vi "dirtyVision.vi"(11 "Plugin Info":T1) -> ()   [LabVIEW 2016]
uses:
  General/CorePluginInfo.ctl
panel:
  out "Frame Rate":dbl
  out "Image Out":T2(plugin-control)
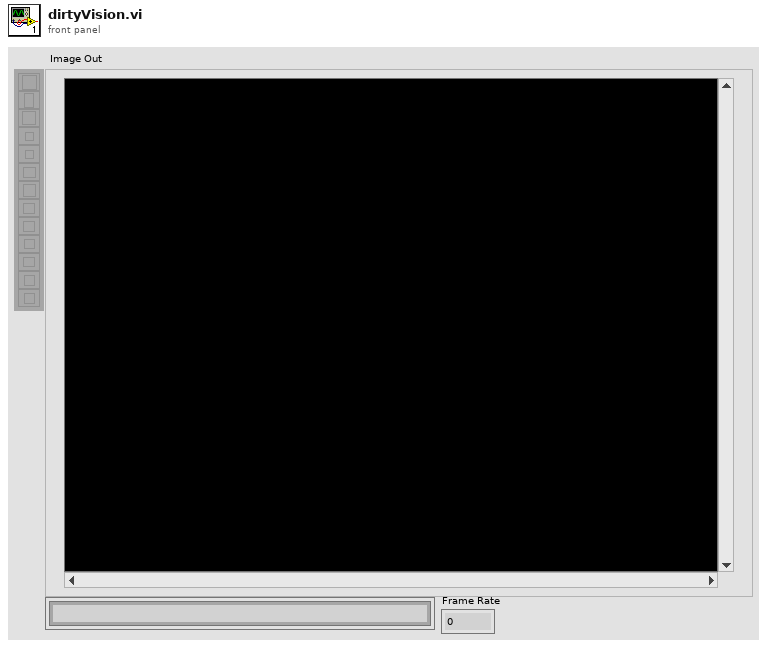
[diagram p1: front panel]
types:
  T1 = typedef "CorePluginInfo.ctl" = cluster{"Notifiers":cluster{"Robot IP Notifier":refnum<notifier>, "Window Mode Notifier":refnum<notifier>, "Stop Notifier":refnum<notifier>}}
  T2 = typedef "IMAQ Image.ctl" = refnum<image>
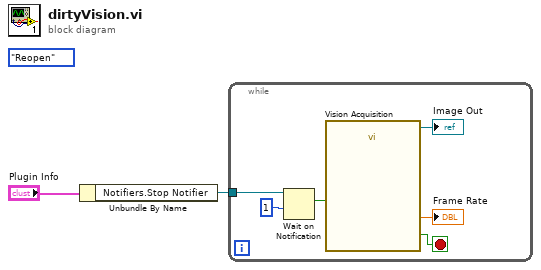
[diagram p0: block diagram]
diagram:
  (unwired) enum16{"Read", "Reopen", "Close"}."Reopen" ("Operation")
  n1 = Unbundle By Name("Plugin Info") -> ("Notifiers.Stop Notifier"=w1:refnum<notifier>)
  n2 = while {
    tunnel: w1 -> [w5]
    stop <- w7 stop-if-true
    n3 = Wait on Notification(notifier=w5, timeout in ms (-1)=1) -> (notification=w3:bool)  [unwired: 2 in, 3 out]
    n4 = call "Vision Acquisition"("Stop (F)"=w3) -> ("Image Out"=→"Image Out":T2, "Frame Rate"=→"Frame Rate":dbl, "Stopped"=w7:bool)  [unwired: 23 in, 1 out]
  }
